vi "test.vi"() -> ()   [LabVIEW 2012]
panel:
  out "Camera Handle 2":u32
  out "error out":errorcluster
  in  "Camera Handle":u32
  in  "stop":bool
  in  "error in (no error)":errorcluster
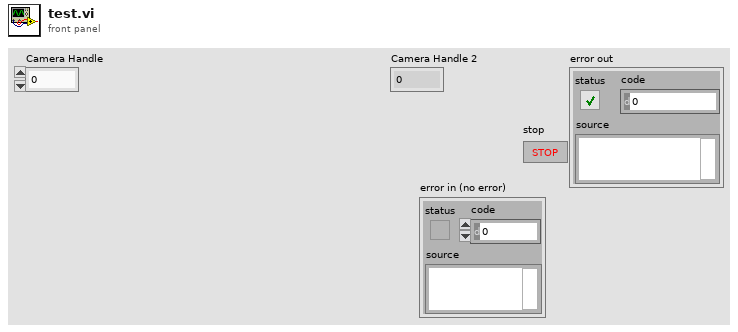
[diagram p1: front panel]
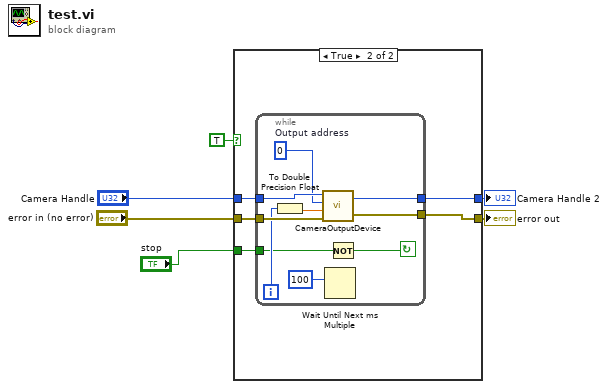
[diagram p0: block diagram]
diagram:
  n1 = case shown="True" TRUE {
    tunnel: "Camera Handle" -> [w8 w13]
    tunnel: "error in (no error)" -> [w7 w12]
    tunnel: [w7 w11] -> w4
    tunnel: [w8 w10] -> w3
    tunnel: "stop" -> [_ w9]
    frame False {
    }
    frame True {
      n2 = while {
        tunnel: w12 -> [w23]
        tunnel: w13 -> [w22]
        tunnel: [w21] -> w10
        tunnel: [w20] -> w11
        tunnel: w9 -> [w14]
        i -> [w18]
        stop <- w15 continue-if-true
        w16 = 0  # Output address
        n3 = To Double Precision Float(number=w18) -> (double precision float=w17:dbl)
        n4 = call "CameraOutputDevice.vi"("error in"=w23, "Output value"=w17, "Output Address"=w16, "Camera Handle"=w22) -> ("error out"=w20:errorcluster, "Camera Handle"=w21:u32)
        n5 = Wait Until Next ms Multiple(millisecond multiple=100) -> ()  [unwired: 1 out]
        n6 = Not(x=w14) -> (.not. x?=w15:bool)
      }
    }
  }
  "error out" <- w4
  "Camera Handle 2" <- w3
